vi "Define 1D Heat PDE Domain.vi"(0 "PDE in":refnum<class "NI_PDE.lvclass">, 5 "T":T2={"initial t"=0.0, "final t"=1.0, "# of t-points"=11}, 7 "X":T1={"start x"=0.0, "end x"=1.0, "# of x-points"=11}, 11 "error in (no error)":errorcluster) -> (4 "PDE out":refnum<class "NI_PDE.lvclass">, 15 "error out":errorcluster)   [LabVIEW 2020, in "NI_PDE.lvlib"]
doc: "Defines the domain where you solve the partial differential equation. You must manually select the polymorphic instance to use."
uses:
  <vilib>/gmath/NI_PDE.lvlib
  <vilib>/gmath/pde.llb/PDEClass/NI_PDE.lvclass
  <vilib>/gmath/pde.llb/PDEClass/PDE_Heat_1D/NI_PDE_Heat_1D.lvclass
  e:/builds/penguin/labview/branches/2020/dev/dist/vi.lib/gmath/pde.llb/PDEClass/NI_PDE.lvclass
  <vilib>/gmath/pde.llb/DomainClass/Domain_Evolut_1D/NI_Domain_Evolut_1D.lvclass
  e:/builds/penguin/labview/branches/2020/dev/dist/vi.lib/gmath/pde.llb/DomainClass/NI_Domain.lvclass
  <vilib>/gmath/pde.llb/DomainClass/Domain_Evolut_1D/Domain Data.ctl
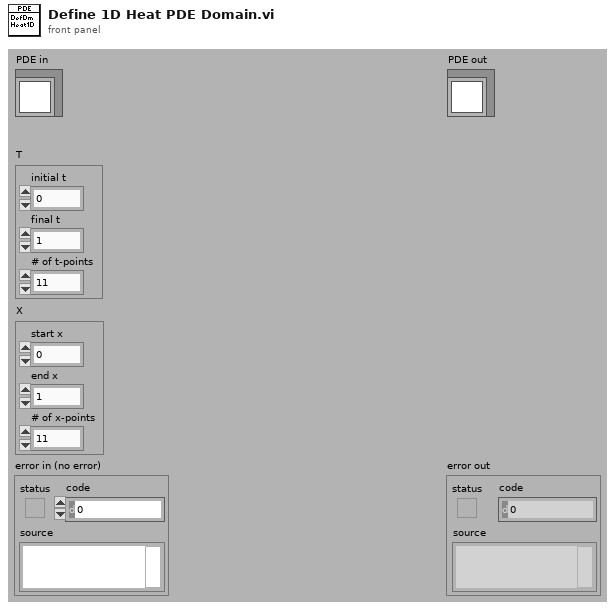
[diagram p1: front panel]
types:
  T1 = cluster{"start x":dbl, "end x":dbl, "# of x-points":i32}
  T2 = cluster{"initial t":dbl, "final t":dbl, "# of t-points":i32}
  T3 = typedef "NI_PDE.lvlib/NI_Domain_Evolut_1D.lvclass/Domain Data.ctl" = cluster{"T":cluster{"initial t":dbl, "final t":dbl, "# of t-points":i32}, "X":cluster{"start x":dbl, "end x":dbl, "# of x-points":i32}}
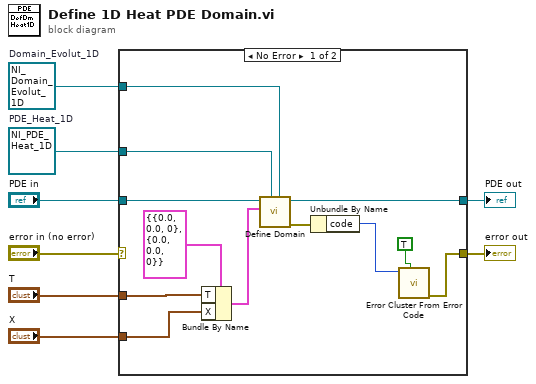
[diagram p0: block diagram]
diagram:
  w1 = refnum<class "NI_Domain_Evolut_1D.lvclass"> refnum  # Domain_Evolut_1D
  w2 = refnum<class "NI_PDE_Heat_1D.lvclass"> refnum  # PDE_Heat_1D
  n1 = case shown="No Error" "error in (no error)" {
    selector: "error in (no error)" -> [_ w22]
    tunnel: [w17 w21] -> w8
    tunnel: "PDE in" -> [w15 w21]
    tunnel: "T" -> [w13 _]
    tunnel: "X" -> [w12 _]
    tunnel: [w18 w22] -> w4
    tunnel: w2 -> [w10 _]
    tunnel: w1 -> [w9 _]
    frame No Error {
      n2 = Bundle By Name(cluster=T3 {"T"={"initial t"=0.0, "final t"=0.0, "# of t-points"=0}, "X"={"start x"=0.0, "end x"=0.0, "# of x-points"=0}} ("domain data"), "T"=w13, "X"=w12) -> (w11:T3)
      n3 = call <vilib>:"Define Domain.vi"("target Domain"=w9, "target PDE"=w10, "domain"=w11, "PDE in"=w15) -> ("error out"=w16:errorcluster, "PDE out"=w17:refnum<class "NI_PDE.lvclass">)  [unwired: 1 in, 5 out]
      n4 = Unbundle By Name(w16) -> ("code"=w20:i32)
      n5 = call <vilib>:"Error Cluster From Error Code.vi"("show call chain? (False)"=TRUE, "error code (0)"=w20) -> ("error out"=w18:errorcluster)  [unwired: 1 in, 6 out]
    }
    frame Error {
    }
  }
  "PDE out" <- w8
  "error out" <- w4
